vi "Memory.Digital.Selection.vi"(11 "memory":refnum<k21>="Digital Pattern Gen Memory 0") -> (3 "memory":refnum<k21>="Digital Pattern Gen Memory 0")   [LabVIEW 2019, in "FPGA Wizard Templates.lvlib"]
uses:
  FPGA Wizard Templates.lvlib
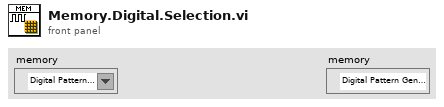
[diagram p1: front panel]
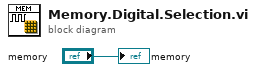
[diagram p0: block diagram]
diagram:
  "memory" <- "memory"
